vi "API Cleanup Directory.vi"() -> ()   [LabVIEW 2017]
uses:
  <vilib>/Utility/QuickDropSupport/QuickDrop Plugin Data ver1.ctl
  Users/Tanner Blair/Documents/LabVIEW Data/Quick Drop Plugins/Align To Connector Pane Sub VIs/Align To Connector.lvlib
panel:
  in  "BD Cleanup":bool
  in  "VI path":path=path "C:/github/data-sharing-framework/Source/Configuration API/Classes"
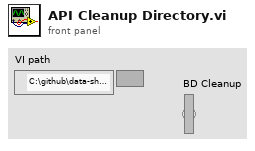
[diagram p1: front panel]
types:
  T1 = typedef "QuickDrop Plugin Data ver1.ctl" = cluster{"FP.IsFrontMost?":bool, "Project VI Path":path, "Palette Object Name":string}
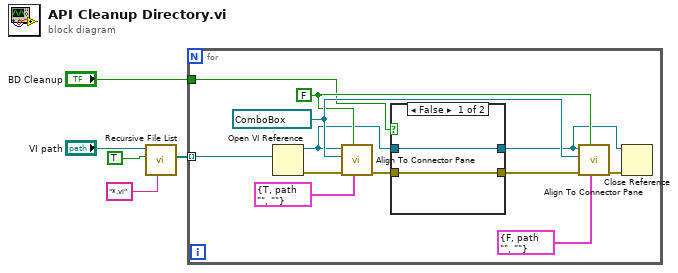
[diagram p0: block diagram]
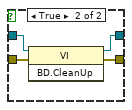
[diagram p2: hidden frame]
diagram:
  n1 = call <vilib>:"Recursive File List.vi"("pattern"="*.vi", "Treat LLBs as Folders?"=TRUE ("Continue Recursing on Error? (F)"), "Folder Path"="VI path") -> ("All Files in Dir"=w3:path[])  [unwired: 4 in, 4 out]
  n2 = for {
    tunnel: w3 -> [w17] mode=indexing
    tunnel: "BD Cleanup" -> [w6]
    w13 = FALSE ("Shift Pressed?")
    w14 = refnum<vi> refnum ("QD Combo Box Ref")
    n3 = Open VI Reference(vi path=w17) -> (vi reference=w9:refnum<vi>, error out=w16:errorcluster)  [unwired: 5 in]
    n4 = call "Align To Connector Pane.vi"("Variant in"=T1 {"FP.IsFrontMost?"=TRUE, "Project VI Path"=path "", "Palette Object Name"=""} ("Quick Drop Plugin Data"), "Shift Pressed?"=w13, "error in (no error)"=w16, "QD Combo Box Ref"=w14, "QD Launch VI Ref"=w9) -> ("error out"=w12:errorcluster)  [unwired: 5 in, 1 out]
    n5 = case shown="False" w6 {
      tunnel: w12 -> [w18 w23]
      tunnel: [w18 w22] -> w10
      tunnel: w9 -> [w19 w21]
      tunnel: [w19 w20] -> w8
      frame False {
      }
      frame True {
        n6 = invoke class="VI" method="BD.CleanUp"(reference=w21, error in=w23) -> (reference out=w20:refnum<vi>, error out=w22:errorcluster)  [unwired: 1 in, 1 out]
      }
    }
    n7 = call "Align To Connector Pane.vi"("Variant in"=T1 {"FP.IsFrontMost?"=FALSE, "Project VI Path"=path "", "Palette Object Name"=""} ("Quick Drop Plugin Data"), "Shift Pressed?"=w13, "error in (no error)"=w10, "QD Combo Box Ref"=w14, "QD Launch VI Ref"=w8) -> ("error out"=w7:errorcluster)  [unwired: 5 in, 1 out]
    n8 = Close Reference(reference=w8, error in (no error)=w7) -> ()  [unwired: 1 out]
  }
